vi "PDC_GetRecordRateList.vi"(8 "error in (no error)":errorcluster, 10 "ChildNo":u32, 11 "DeviceNo":u32) -> (0 "error out":errorcluster, 1 "List":u32[](array[numeric]), 2 "Size":u32, 3 "ReturnValue":u32, 4 "ErrorCode":u32)   [LabVIEW 2015]
doc: "This VI retrieves the list of recording speeds that can be set in the specified child device."
uses:
  PDCLIB.dll
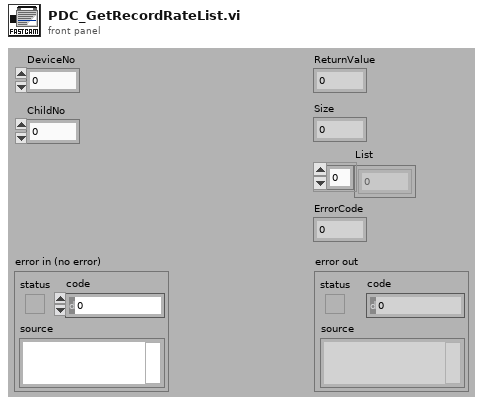
[diagram p1: front panel]
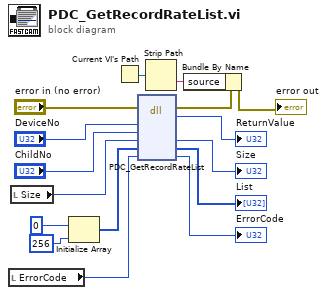
[diagram p0: block diagram]
diagram:
  n1 = local read "ErrorCode"() -> (w13:u32)
  n2 = local read "Size"() -> (w10:u32)
  n3 = Initialize Array(u32 0, 256 ("dimension size")) -> (w9:u32[])
  n4 = Current VI's Path() -> (path=w4:path)
  n5 = dll-call lib="PDCLIB.dll" fn="PDC_GetRecordRateList"(error in="error in (no error)", "nDeviceNo"="DeviceNo", "nChildNo"="ChildNo", "pSize"=w10, "pList"=w9, "pErrorCode"=w13) -> (error out=w3:errorcluster, "return type"=→"ReturnValue":u32, "pSize"=→"Size":u32, "pList"=→"List":u32[], "pErrorCode"=→"ErrorCode":u32)  [unwired: 4 in, 1 out]
  n6 = Strip Path(path=w4) -> (name=w5:string)  [unwired: 1 out]
  n7 = Bundle By Name(cluster=w3, "source"=w5) -> (→"error out":errorcluster)
